vi "Main - Closed Loop Basic _3.vi"() -> ()   [LabVIEW 2017]
uses:
  Pitch Array 1.ctl
  <vilib>/Analysis/coordinate.llb/Angle Units.ctl
  <vilib>/Analysis/coordinate.llb/Angle Range (Degree).ctl
  <vilib>/Analysis/coordinate.llb/Wrap Angle (scalar).vi
  <vilib>/Utility/file.llb/Read Delimited Spreadsheet (DBL).vi
  <vilib>/Analysis/NI_AAL_Angle.lvlib
panel:
  out "Pitch Sensor \nCalibration Data":dbl[][](array[numeric])
  in  "Base Path For MATLAB Controller Parameter Files":path=path "MATLAB Parameter File Directory"
  out "Travel Ref (Absolute)":dbl=6.278649578908132 format="%.1f"
  out "Pitch F/B":dbl(slide)=6.367486645190397 scale=-85.0..85.0
  out "Run Time (s)":u32=182
  out "Pitch Est":dbl(slide)=6.367244037580416 scale=-85.0..85.0
  out "Elevation Est":dbl(slide)=6.884551861272796 scale=-45.0..45.0
  out "Travel Est (Absolute)":dbl=-19.800319506146298 format="%.1f"
  out "Fan Control":dbl[](array[numeric])=[8.156223656379174, 7.8664338572886825] format="%#.1f"
  out "Step Size (ms)":u32=15
  out "Fan B":dbl(slide)=7.8664338572886825 scale=0.0..10.0
  out "Fan A":dbl(slide)=8.156223656379174 scale=0.0..10.0
  in  "Travel Ref":dbl(knob)=6.278649578908132 scale=0.0..360.0
  in  "Elevation Ref":dbl(slide)=6.428571428571431 scale=-40.0..25.0
  out "Elevation F/B":dbl(slide)=6.884194681467489 scale=-45.0..45.0
  in  "stop":bool
  out "Travel F/B (Absolute)":dbl=-19.8 format="%.1f"
  out "Travel Angle":cluster{dbl, dbl, dbl}(knob)={340.2, 340.19967871200294, 6.278649578908132} scale=0.0..360.0
  # "F/B"
  # "Est"
  # "Ref"
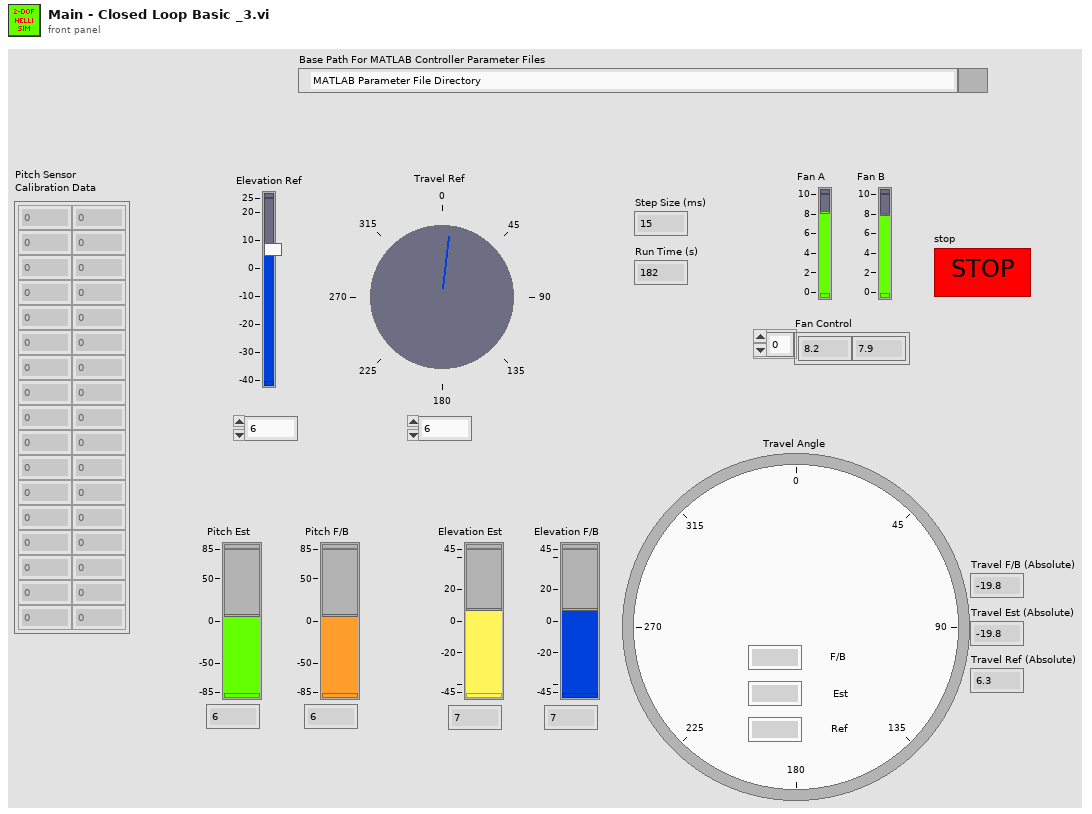
[diagram p1: front panel]
types:
  T1 = typedef "Pitch Array 1.ctl" = cluster{"Array":dbl[][], "Operation":bool}
  T2 = cluster{"AI Task":refnum<k21>, "Ctr0 Task":refnum<k21>, "Ao Task":refnum<k21>, "DO Task":refnum<k21>}
  T3 = typedef "NI_Matrix.lvlib/RealMatrix.ctl" = dbl[][]
  T4 = typedef "NI_LinSys_Model Typedefs.lvlib/CD State Space Model (MIMO).ctl" = cluster{"properties":T5, "A":dbl[][], "B":dbl[][], "C":dbl[][], "D":dbl[][], "StateNames":string[], "Transport Delay":dbl[][]}
  T5 = typedef "NI_LinSys_Model Typedefs.lvlib/CD General Elements.ctl" = cluster{"Model name":string, "Input names":string[], "Output names":string[], "Input Delays":dbl[], "Output Delays":dbl[], "Sampling Time":dbl, "Notes":string}
  T6 = cluster{"L1":dbl, "L2":dbl, "L3":dbl, "Jp":dbl, "Jt":dbl, "Je":dbl, "m1":dbl, "m2":dbl, "g":dbl, "Ts":dbl, "Fan Thrust":dbl[][], "U_e":dbl[], "Kdi Matrix":T3, "Kd Matrix":T3, "DT KF State-Space Model":T4, "Cr Matrix":T3}
  T7 = typedef "NI_AAL_Angle.lvlib/Angle Range (Degree).ctl" = u16
  T8 = typedef "NI_AAL_Angle.lvlib/Angle Units.ctl" = i32
  T9 = cluster{"angle out":dbl, "angle out":dbl, "angle out":dbl}
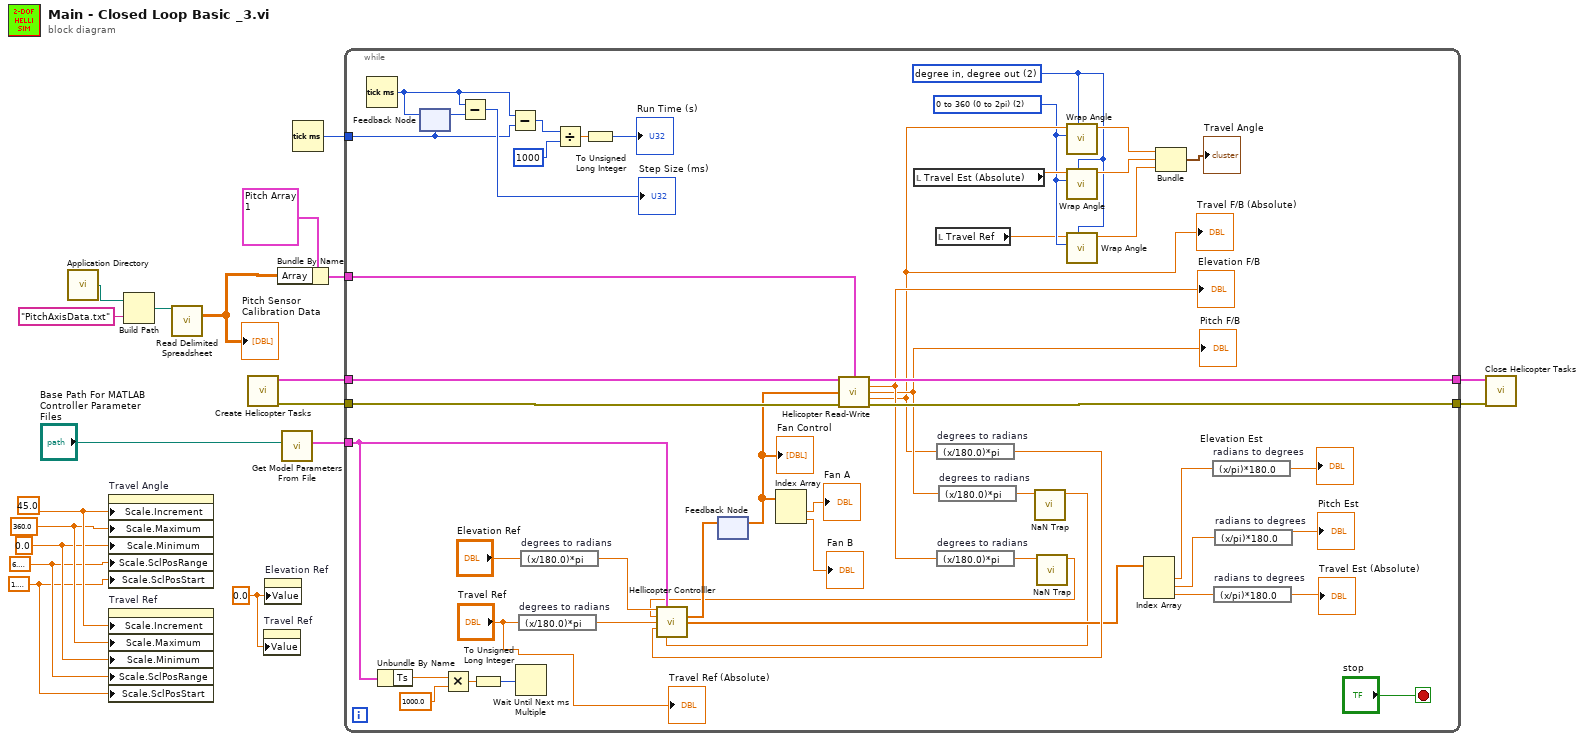
[diagram p0: block diagram]
diagram:
  w6 = 1.5707963267948966
  w9 = 360.0 ("Scale.Range:Maximum")
  w10 = 45.0 ("Scale.Range:Increment")
  w7 = 6.283185307179586
  w8 = 0.0 ("Scale.Scale Position:Start")
  w15 = 0.0 ("ElevRef")
  n1 = call <vilib>:"Application Directory.vi"() -> ("Application Directory"=w3:path)
  n2 = property on="Travel Angle" class="Knob (strict)"("Scale.Increment"=w10, "Scale.Maximum"=w9, "Scale.Minimum"=w8, "Scale.SclPosRange"=w7, "Scale.SclPosStart"=w6) -> ()  [unwired: 2 in, 2 out]
  n3 = property on="Travel Ref" class="Knob (strict)"("Scale.Increment"=w10, "Scale.Maximum"=w9, "Scale.Minimum"=w8, "Scale.SclPosRange"=w7, "Scale.SclPosStart"=w6) -> ()  [unwired: 2 in, 2 out]
  n4 = Build Path(base path=w3, name or relative path="PitchAxisData.txt") -> (appended path=w1:path)
  n5 = call-poly <vilib>:"Read Delimited Spreadsheet.vi"("file path (dialog if empty)"=w1) -> ("all rows"=w2:dbl[][])  [unwired: 9 in, 5 out]
  "Pitch Sensor \nCalibration Data" <- w2
  n6 = call "Create Helicopter Tasks.vi"() -> ("Error Out"=w14:errorcluster, "Hellicopter Tasks Output"=w13:T2)  [unwired: 6 in]
  n7 = property on="Travel Ref" class="Knob (strict)"("Value"=w15) -> ()  [unwired: 2 in, 2 out]
  n8 = property on="Elevation Ref" class="Slide (strict)"("Value"=w15) -> ()  [unwired: 2 in, 2 out]
  n9 = Bundle By Name(cluster=T1 {"Array"=[[80.0, 0.9, 1.0, 1.0, 1.0, 1.0, 1.0, 1.0, 1.0], [70.0, 0.96, 0.0, 0.0, 0.0, 0.0, 0.0, 0.0, 0.0], [60.0, 1.08, 0.0, 0.0, 0.0, 0.0, 0.0, 0.0, 0.0], [50.0, 1.25, 0.0, 0.0, 0.0, 0.0, 0.0, 0.0, 0.0], [40.0, 1.44, 0.0, 0.0, 0.0, 0.0, 0.0, 0.0, 0.0], [30.0, 1.68, 0.0, 0.0, 0.0, 0.0, 0.0, 0.0, 0.0], [20.0, 1.91, 0.0, 0.0, 0.0, 0.0, 0.0, 0.0, 0.0], [10.0, 2.19, 0.0, 0.0, 0.0, 0.0, 0.0, 0.0, 0.0], [0.0, 2.47, 0.0, 0.0, 0.0, 0.0, 0.0, 0.0, 0.0], [-10.0, 2.73, 0.0, 0.0, 0.0, 0.0, 0.0, 0.0, 0.0], [-20.0, 3.01, 0.0, 0.0, 0.0, 0.0, 0.0, 0.0, 0.0], [-30.0, 3.3, 0.0, 0.0, 0.0, 0.0, 0.0, 0.0, 0.0], [-40.0, 3.5, 0.0, 0.0, 0.0, 0.0, 0.0, 0.0, 0.0], [-50.0, 3.72, 0.0, 0.0, 0.0, 0.0, 0.0, 0.0, 0.0], [-60.0, 3.92, 0.0, 0.0, 0.0, 0.0, 0.0, 0.0, 0.0], [-70.0, 4.05, 0.0, 0.0, 0.0, 0.0, 0.0, 0.0, 0.0], [-80.0, 4.11, 0.0, 0.0, 0.0, 0.0, 0.0, 0.0, 0.0]], "Operation"=FALSE} ("Pitch Calib"), "Array"=w2) -> (w12:T1)
  n10 = call "Get Model Parameters From File.vi"("Base Path For Model"="Base Path For MATLAB Controller Parameter Files") -> ("Model Parameters"=w19:T6)  [unwired: 9 in, 1 out]
  n11 = Tick Count (ms)() -> (millisecond timer value=w18:u32)
  n12 = while {
    tunnel: w19 -> [w65]
    tunnel: w18 -> [w45]
    tunnel: [w40] -> w17
    tunnel: [w39] -> w16
    tunnel: w13 -> [w42]
    tunnel: w14 -> [w41]
    tunnel: w12 -> [w31]
    stop <- "stop" stop-if-true
    w23 = T7 2 items=["none", "-180 to 180 (-pi to pi)", "0 to 360 (0 to 2pi)"] ("angle range")
    w24 = T8 2 items=["radian in, radian out", "radian in, degree out", "degree in, degree out", "degree in, radian out"] ("angle units")
    n13 = Tick Count (ms)() -> (millisecond timer value=w46:u32)
    n14 = Unbundle By Name(w65) -> ("Ts"=w67:dbl)
    n15 = feedback-in #1(w46) -> ()
    n16 = feedback #1(w45) -> (w66:u32)
    n17 = Multiply(x=w67, y=1000.0) -> (x*y=w68:dbl)
    n18 = Subtract(x=w46, y=w66) -> (x-y=→"Step Size (ms)":u32)
    n19 = To Unsigned Long Integer(number=w68) -> (unsigned 32bit integer=w60:u32)
    n20 = Subtract(x=w46, y=w45) -> (x-y=w44:u32)
    n21 = Wait Until Next ms Multiple(millisecond multiple=w60) -> ()  [unwired: 1 out]
    n22 = expression code="(x/180.0)*pi" "degrees to radians"("Travel Ref") -> (w63:dbl)
    n23 = expression code="(x/180.0)*pi" "degrees to radians"("Elevation Ref") -> (w64:dbl)
    n24 = Divide(x=w44, y=u32 1000) -> (x/y=w47:dbl)
    n25 = To Unsigned Long Integer(number=w47) -> (unsigned 32bit integer=→"Run Time (s)":u32)
    n26 = feedback #2() -> (w32:dbl[])  [unwired: 1 in]
    "Fan Control" <- w32
    n27 = Index Array(array=w32) -> (element #1=→"Fan A":dbl, element #2=→"Fan B":dbl)  [unwired: 2 in]
    n28 = call "Helicopter Read-Write.vi"("Hellicopter Tasks Input"=w42, "Pitch Calib"=w31, "Fan Input"=w32, "Error In"=w41) -> ("Hellicopter Tasks Output"=w40:T2, "Elevation"=w38:dbl, "Pitch"=w37:dbl, "Travel"=w25:dbl, "Error Out"=w39:errorcluster)  [unwired: 7 in]
    "Travel F/B (Absolute)" <- w25
    "Elevation F/B" <- w38
    "Pitch F/B" <- w37
    n29 = local read "Travel Est (Absolute)"() -> (w26:dbl)
    n30 = local read "Travel Ref"() -> (w22:dbl)
    n31 = expression code="(x/180.0)*pi" "degrees to radians"(w25) -> (w57:dbl)
    n32 = expression code="(x/180.0)*pi" "degrees to radians"(w38) -> (w50:dbl)
    n33 = expression code="(x/180.0)*pi" "degrees to radians"(w37) -> (w30:dbl)
    n34 = call "NaN Trap.vi"("Elevation in"=w30) -> ("Elevation out"=w29:dbl)  [unwired: 9 in, 1 out]
    n35 = call "NaN Trap.vi"("Elevation in"=w50) -> ("Elevation out"=w56:dbl)  [unwired: 9 in, 1 out]
    n36 = call "Hellicopter Controlller.vi"("ElevRef"=w64, "Model Parameters"=w65, "ElevFB"=w56, "TravRef"=w63, "TravFB"=w57, "PitchFB"=w29) -> ("Fan Control (Bounded)"=w58:dbl[], "KF Output"=w33:dbl[])  [unwired: 5 in, 3 out]
    n37 = feedback-in #2(w58) -> ()
    n38 = call-poly <vilib>:"Wrap Angle.vi"("angle units"=w24, "angle range"=w23, "angle in"=w25) -> ("angle out"=w27:dbl)  [unwired: 7 in, 1 out]
    n39 = call-poly <vilib>:"Wrap Angle.vi"("angle units"=w24, "angle range"=w23, "angle in"=w26) -> ("angle out"=w28:dbl)  [unwired: 7 in, 1 out]
    n40 = call-poly <vilib>:"Wrap Angle.vi"("angle units"=w24, "angle range"=w23, "angle in"=w22) -> ("angle out"=w21:dbl)  [unwired: 7 in, 1 out]
    n41 = Index Array(array=w33) -> (element #1=w53:dbl, element #2=w34:dbl, element #3=w35:dbl)  [unwired: 3 in]
    n42 = Bundle("angle out"=w27, "angle out"=w28, "angle out"=w21) -> (→"Travel Angle":T9)  [unwired: 1 in]
    n43 = expression code="(x/pi)*180.0" "radians to degrees"(w53) -> (→"Elevation Est":dbl)
    n44 = expression code="(x/pi)*180.0" "radians to degrees"(w35) -> (→"Travel Est (Absolute)":dbl)
    n45 = expression code="(x/pi)*180.0" "radians to degrees"(w34) -> (→"Pitch Est":dbl)
    "Travel Ref (Absolute)" <- "Travel Ref"
  }
  n46 = call "Close Helicopter Tasks.vi"("Error In"=w16, "Hellicopter Tasks Input 2"=w17) -> ()  [unwired: 9 in, 1 out]
